vi "runImageViewer.vi"(9 "remote port":u16=6342, 10 "remote address":string="localhost") -> ()   [LabVIEW 2009, in "run.lvlib"]
uses:
  run.lvlib
  Viewers/ImageStreamViewer/ImageStreamViewer.lvclass
  Viewers/ImageStreamDecoder/ImageStreamDecoder.lvclass
  HWController/Network Controllers/NetworkClient/NetworkServer.lvclass
  Tools/Filing/FileNeologist/FileNeologist.lvclass
panel:
  # "run"
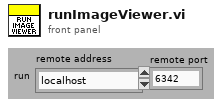
[diagram p1: front panel]
types:
  T1 = enum32{"Invalid", "Standard", "Closed", "Hidden", "Minimized", "Maximized"}
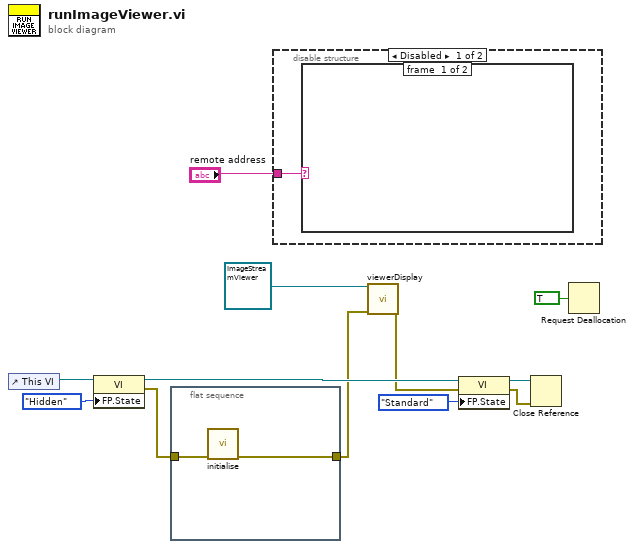
[diagram p0: block diagram]
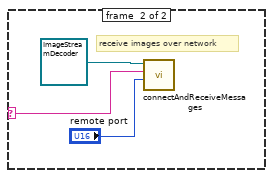
[diagram p2: hidden frame]
diagram:
  n1 = control-ref of="This VI"() -> (w10:refnum<vi>)
  n2 = property class="VI"(reference=w10, "FP.State"=T1."Hidden" ("Front Panel Window:State")) -> (reference out=w8:refnum<vi>, error out=w2:errorcluster)  [unwired: 1 in]
  n3 = flat-sequence {
    tunnel: w2 -> [w14]
    tunnel: [w13] -> w1
    frame #0 {
      n4 = call "initialise.vi"("error in (no error)"=w14) -> ("error out"=w13:errorcluster)  [unwired: 9 in, 1 out]
    }
  }
  n5 = disable-structure shown="Disabled" {
    disable-tunnel: "remote address" -> [w15 _]
    frame #0 {
      n6 = case shown="Default" w15 {
        selector: w15 -> [_ w16]
        frame #0 {
        }
        frame #1 {
          # "receive images over network"
          n7 = call "connectAndReceiveMessages.vi"("remote port"="remote port", "remote address"=w16, "NetworkServer in"=refnum<class "ImageStreamDecoder.lvclass"> refnum ("Hardware:HWControllers.lvlib:ImageStreamDecoder.lvclass")) -> ()  [unwired: 7 in, 2 out]
        }
      }
    }
    frame #1 {
    }
  }
  n8 = call "viewerDisplay.vi"("error in (no error)"=w1, "ImageStreamViewer in"=refnum<class "ImageStreamViewer.lvclass"> refnum) -> ("error out"=w7:errorcluster)  [unwired: 8 in, 1 out]
  n9 = property class="VI"(reference=w8, error in=w7, "FP.State"=T1."Standard" ("Front Panel Window:State")) -> (reference out=w4:refnum<vi>, error out=w5:errorcluster)
  n10 = Close Reference(reference=w4, error in (no error)=w5) -> ()  [unwired: 1 out]
  n11 = Request Deallocation(TRUE ("flag")) -> ()
